vi "IsTimerDoneSubVI.vi"(8 "End Time (Seconds)":dbl, 11 "Get Time (Seconds)":dbl) -> (3 "Time Done":bool)   [LabVIEW 2019]
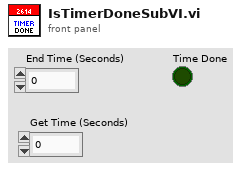
[diagram p1: front panel]
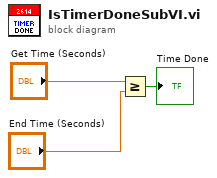
[diagram p0: block diagram]
diagram:
  n1 = Greater Or Equal?(x="Get Time (Seconds)", y="End Time (Seconds)") -> (x >= y?=→"Time Done":bool)
